vi "PH_PILS.PC _Laserpower.vi"(0 "i ref in":refnum<vi>, 2 "serviceName":string, 3 "Value":i32, 5 "error IO":errorcluster) -> (14 "i ref out":refnum<vi>, 19 "error out":errorcluster)   [LabVIEW 2014, in "PH_PILS.lvlib"]
doc: "This VI sets the incoming tag values to own attributes."
uses:
  PH_PILS.lvlib
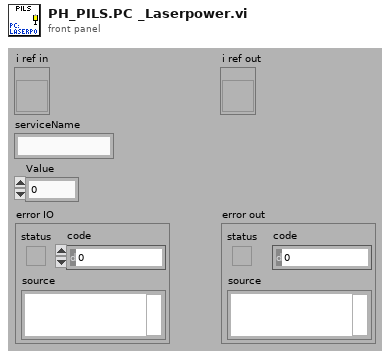
[diagram p1: front panel]
types:
  T1 = typedef "PH_PILS.lvlib/PH_PILS.i attribute.ctl" = cluster{"Boolean":cluster{"GUI Ref":refnum<vi>, "Status":i32}[], "GUI Refs Exp. Shutters":cluster{"1":refnum<vi>, "2":refnum<vi>, "3":refnum<vi>, "4":refnum<vi>}, "Tristate2Run GUI Refs":refnum<vi>[], "EO-Likes":cluster{"GUI Ref":refnum<vi>, "Status":i32}[], "Operation Mode":cluster{"Operation Mode":T2, "GUI":cluster{"Ref State":refnum<vi>, "Ref":refnum<vi>}, "Servicemode":cluster{"Tagname":string, "Status":i32}, "Labormode":cluster{"Tagname":string, "Status":i32}, "Searchmode":cluster{"Tagname":string, "Status":i32}, "Shotmode":cluster{"Tagname":string, "Status":i32}}, "Submode":cluster{"Submode":T3, "GUI":cluster{"Ref State":refnum<vi>, "Ref":refnum<vi>}, "Submode":cluster{"Tagname":string, "Status":i32}}, "Experiment":cluster{"Experiment":enum16{"unknown", "intern", "4 (Z6)", "3", "2", "1"}, "GUI":cluster{"Ref State":refnum<vi>, "Ref":refnum<vi>}, "intern":cluster{"Tagname":string, "Status":i32}, "Exp 4":cluster{"Tagname":string, "Status":i32}, "Exp 3":cluster{"Tagname":string, "Status":i32}, "Exp 2":cluster{"Tagname":string, "Status":i32}, "Exp 1":cluster{"Tagname":string, "Status":i32}}, "TristateNormal":cluster{"GUI Ref":refnum<vi>, "Status":i32}[], "Door Tags":cluster{"GUI Ref":refnum<vi>, "Status":i32}[], "GUIlessTags":cluster{"Name":string, "Status":i32}[], "Beamline GUI Refs":refnum<vi>[], "Special Boolean":cluster{"GUI Ref":refnum<vi>, "Status":i32}[], "Laserpower":cluster{"GUI Ref":refnum<vi>, "Status":i32}[], "Shutter":cluster{"GUI Ref":refnum<vi>, "Status":i32}[], "Tristate EO Like":cluster{"GUI Ref":refnum<vi>, "Status":i32}[], "PP":cluster{"GUI Ref":refnum<vi>, "Status":i32, "Head Ref":refnum<vi>, "Slider Ref":refnum<vi>}[], "Switch Knobs":cluster{"GUI Ref":refnum<vi>, "Status":i32}[], "Latch Knob GUI Refs":refnum<vi>[], "FailureCounter":i32, "Enabled Status":cluster{"Laser":i32, "PreAmp":i32, "MainAmp":i32}, "Mercury":refnum<vi>, "Instance Rods":string, "Logfile":path, "Beckhoff-Instance Internal":string, "Beckhoff-Instance External":string, "Enabling Rights":cluster{"Name":string, "Password":string, "PA?":bool, "MA?":bool, "Exp?":bool}[]}
  T2 = typedef "PH_PILS.lvlib/PH_PILS.Operation Mode.ctl" = enum16{"unknown", "Service", "Labor", "Search", "Shot"}
  T3 = typedef "PH_PILS.lvlib/PH_PILS.Submode.ctl" = enum16{"unknown", "HV-Normal", "HV-Test"}
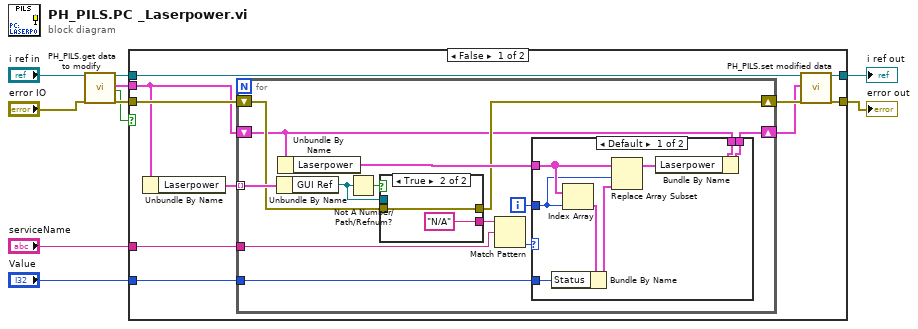
[diagram p0: block diagram]
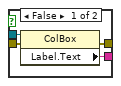
[diagram p3: hidden frame]
diagram:
  n1 = call "PH_PILS.get data to modify.vi"("i ref in"="i ref in", "error in (no error)"="error IO") -> ("i ref out"=w4:refnum<vi>, "i attribute"=w3:T1, "timed out"=w6:bool, "error out"=w7:errorcluster)  [unwired: 14 in]
  n2 = case shown="False" w6 {
    tunnel: w3 -> [w11 _]
    tunnel: w4 -> [w20 w50]
    tunnel: [w19 w50] -> w5
    tunnel: w7 -> [w14 w49]
    tunnel: [w18 w49] -> w8
    tunnel: "Value" -> [w16 _]
    tunnel: "serviceName" -> [w17 _]
    frame False {
      n3 = Unbundle By Name(w11) -> ("Laserpower"=w15:cluster{"GUI Ref":refnum<vi>, "Status":i32}[])
      n4 = for {
        tunnel: w15 -> [w33] mode=indexing
        tunnel: w17 -> [w29]
        tunnel: w16 -> [w26]
        shift-right: [w23] -> w13
        shift-left: w14 -> [w24]
        shift-right: [w22] -> w12
        shift-left: w11 -> [w21]
        i -> [w28]
        n5 = Unbundle By Name(w33) -> ("GUI Ref"=w32:refnum<vi>)
        n6 = Unbundle By Name(w21) -> ("Laserpower"=w25:cluster{"GUI Ref":refnum<vi>, "Status":i32}[])
        n7 = Not A Number/Path/Refnum?(number/path/refnum=w32) -> (NaN/Path/Refnum?=w31:bool)
        n8 = case shown="True" w31 {
          tunnel: w32 -> [w46 _]
          tunnel: [w45 "N/A" ("Label.Text")] -> w30
          tunnel: w24 -> [w44 w47]
          tunnel: [w43 w47] -> w23
          frame False {
            n9 = property class="ColBox"(reference=w46, error in=w44) -> (error out=w43:errorcluster, "Label.Text"=w45:string)  [unwired: 1 out]
          }
          frame True {
          }
        }
        n10 = Match Pattern(string=w30, regular expression=w29) -> (offset past match=w27:i32)  [unwired: 1 in, 3 out]
        n11 = case shown="Default" w27 {
          tunnel: w25 -> [w38 _]
          tunnel: w21 -> [w40 w42]
          tunnel: [w39 w42] -> w22
          tunnel: w26 -> [w37 _]
          tunnel: w28 -> [w34 _]
          frame Default {
            n12 = Index Array(array=w38, index=w34) -> (element=w35:cluster{"GUI Ref":refnum<vi>, "Status":i32})
            n13 = Bundle By Name(cluster=w35, "Status"=w37) -> (w36:cluster{"GUI Ref":refnum<vi>, "Status":i32})
            n14 = Replace Array Subset(array=w38, new element=w36, index=w34) -> (w41:cluster{"GUI Ref":refnum<vi>, "Status":i32}[])
            n15 = Bundle By Name(cluster=w40, "Laserpower"=w41) -> (w39:T1)
          }
          frame -1 {
          }
        }
      }
      n16 = call "PH_PILS.set modified data.vi"("i ref in"=w20, "i attribute"=w12, "error in (no error)"=w13) -> ("i ref out"=w19:refnum<vi>, "error out"=w18:errorcluster)  [unwired: 15 in]
    }
    frame True {
    }
  }
  "error out" <- w8
  "i ref out" <- w5
